vi "Main.vi"(11 "Module Admin":refnum<class "Delacor_lib_QMH_Module Admin.lvclass">) -> ()   [LabVIEW 2026, in "Replay.lvlib"]
doc: "This template is based off of the Queued Message Handler design pattern and the Queued Message Handler project template that ships with LabVIEW.\n\nThe main difference is that the queue is private to this module and communication between modules is performed via Broadcast and Request events.\n\nRequest events are wrapped in public API methods and are handled in the Event Handling Loop (EHL) of this VI. Any module can register for Broadcast events sent by this module. The EHL generates messages based on user interface actions.\n\nThe Message Handling Loop (MHL) processes messages generated by the EHL, or by other messages. The messages are string values, so new messages can be added easily to the Message Cases case structure in the MHL. Each message cluster can also provide an optional value for Message Data, which is a variant that can be converted to whatever message-specific data is required.\n_____\nBased on DQMH Dev Tools: Project Template 7.1.2.1547."
uses:
  Replay.lvlib
  <vilib>/Delacor/Delacor QMH/Libraries/Message Queue_class/Delacor_lib_QMH_Message Queue.lvclass
  Module Data--cluster.ctl
  <vilib>/Utility/miscctls.llb/LVPointTypeDef.ctl
  <vilib>/Delacor/Delacor QMH/Libraries/Message Queue_class/Delacor_lib_QMH_Enqueue Message (Single).vi
  Stop Argument--cluster.ctl
  <vilib>/Delacor/Delacor QMH/Libraries/Module Admin_class/Delacor_lib_QMH_Module Admin.lvclass
  Launcher/Launcher.lvlib
  Replay Helper Loop.ctl
  User Events Metadata.ctl
  <vilib>/Wovalab/Utilities/Helper Loop Periodic Timing/Helper Loop Periodic Timing.lvclass
panel:
  out "error out":errorcluster
  out "Status":string
  in  "Simulate MHL Error":bool
  in  "Simulate EHL Error":bool
  # "Other processes communicate with this Module via its Public API (wrappers for its Request Events).\n\nThis Module communicates with other processes via its Broadcast Events.\nAny process that wants to receive these messages can register for this module's Broadcast events."
  # "This template is for the DQMH framework. See the block diagram for more information on how to use this template."
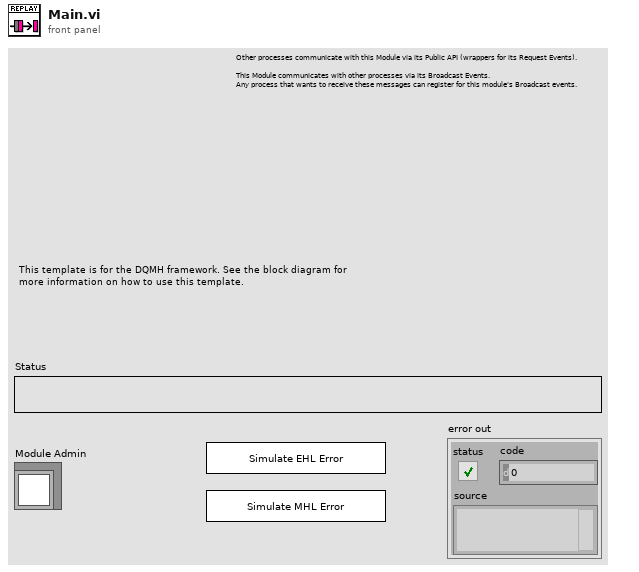
[diagram p1: front panel]
types:
  T1 = typedef "Replay.lvlib/Request Events--cluster.ctl" = cluster{"Stop Module":refnum<user-event>, "Show Panel":refnum<user-event>, "Hide Panel":refnum<user-event>, "Get Module Execution Status":refnum<user-event>, "Show Diagram":refnum<user-event>, "Set Run ID to Replay":refnum<user-event>}
  T2 = typedef "Launcher.lvlib/Broadcast Events--cluster.ctl" = cluster{"Module Did Init":refnum<user-event>, "Status Updated":refnum<user-event>, "Error Reported":refnum<user-event>, "Module Did Stop":refnum<user-event>, "Update Module Execution Status":refnum<user-event>, "Start Capture Detection Loop":refnum<user-event>, "Benchmark Started":refnum<user-event>, "Broadcast number of frames and run ID":refnum<user-event>}
  T3 = typedef "Replay.lvlib/Replay Helper Loop.ctl" = cluster{"Timeout":i32, "Run ID":string, "Replay Array Elements":string[], "User Events Metadata":T4[], "Frame Index":i32}
  T4 = typedef "User Events Metadata.ctl" = cluster{"Cursor Position X":i32, "Cursor Position Y":i32, "Left Button Click":bool, "Right Button Click":bool, "Frame Number":u32}
  T5 = typedef "Replay.lvlib/Module Data--cluster.ctl" = cluster{"Status":string}
  T6 = enum32{"invalid lock state", "Not Locked", "Locked (No Password)", "Password-protected"}
  T7 = typedef "Replay.lvlib/Stop Argument--cluster.ctl" = cluster{"Origin":string, "Exit via Stop Module Req?":bool, "Wait for Module to stop?":bool}
  T8 = typedef "LVPointTypeDef.ctl" = cluster{"Horizontal":i16, "Vertical":i16}
  T9 = enum32{"Invalid", "Standard", "Closed", "Hidden", "Minimized", "Maximized"}
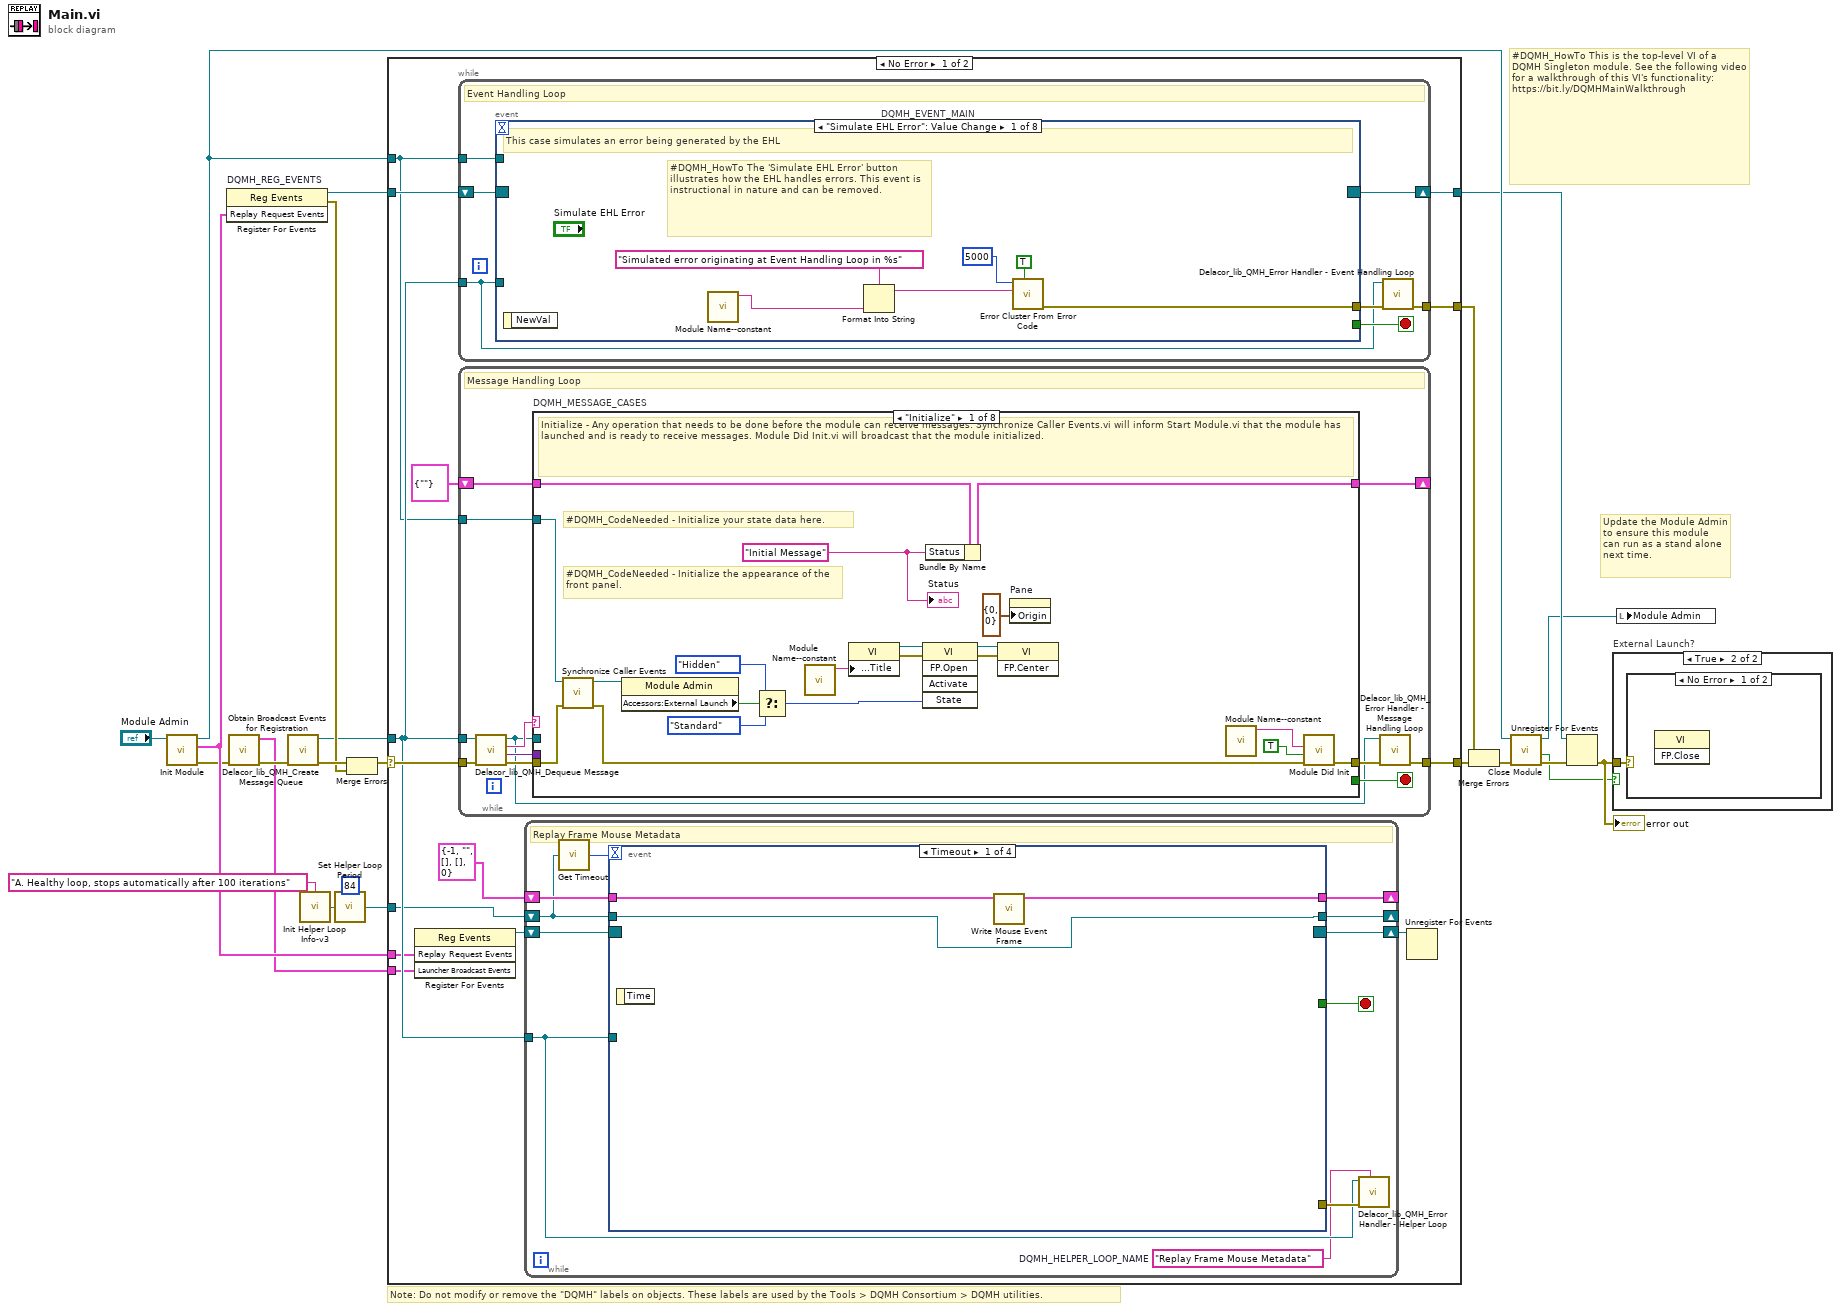
[diagram p0: block diagram]
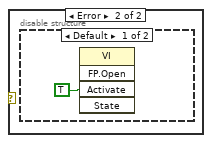
[diagram p3: hidden frame]
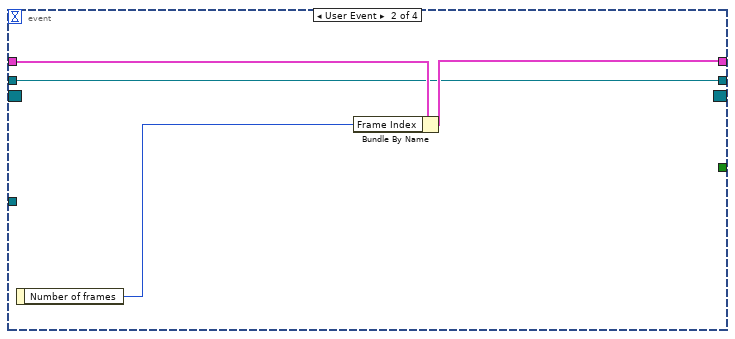
[diagram p5: hidden frame]
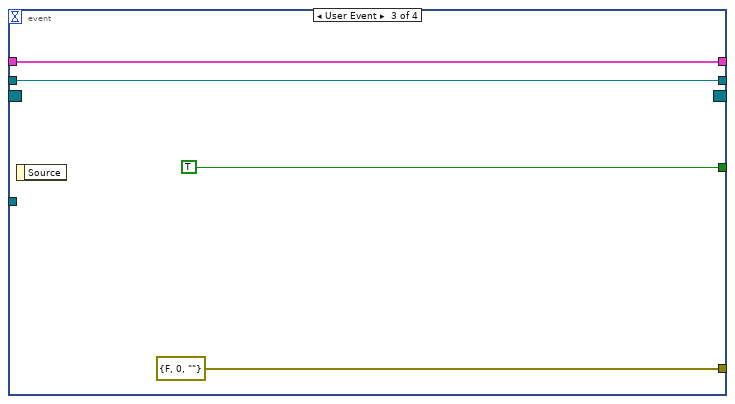
[diagram p6: hidden frame]
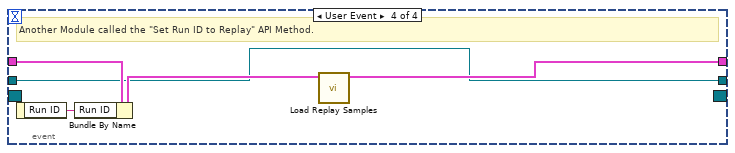
[diagram p7: hidden frame]
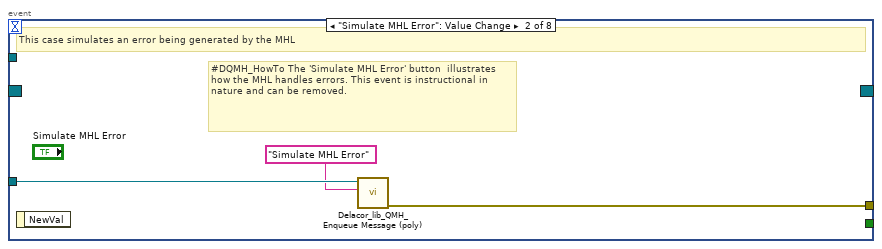
[diagram p8: hidden frame]
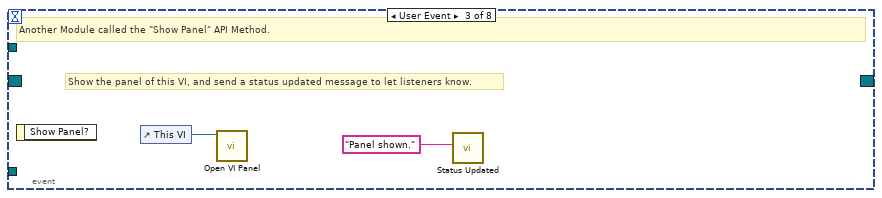
[diagram p9: hidden frame]
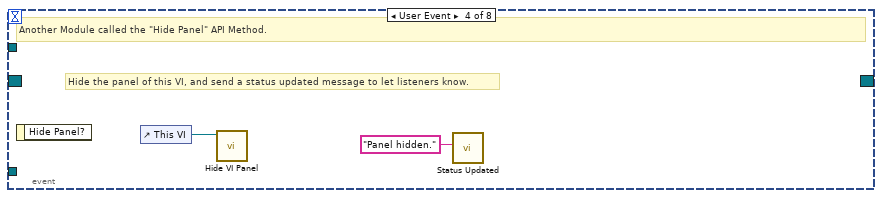
[diagram p10: hidden frame]
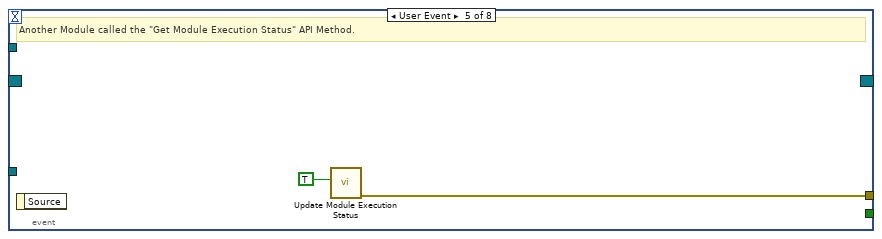
[diagram p11: hidden frame]
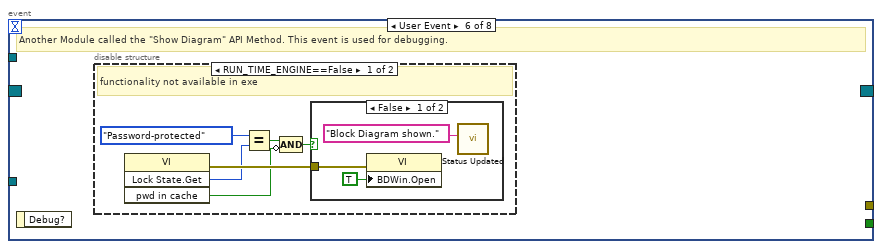
[diagram p12: hidden frame]
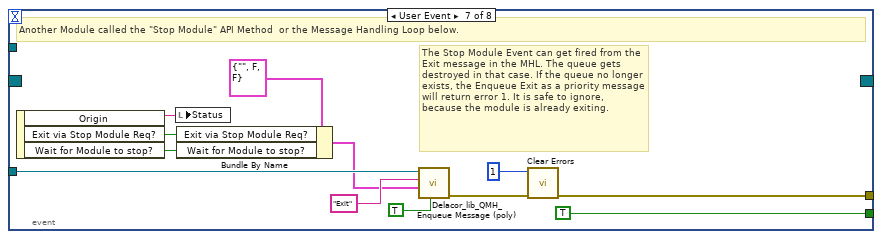
[diagram p15: hidden frame]
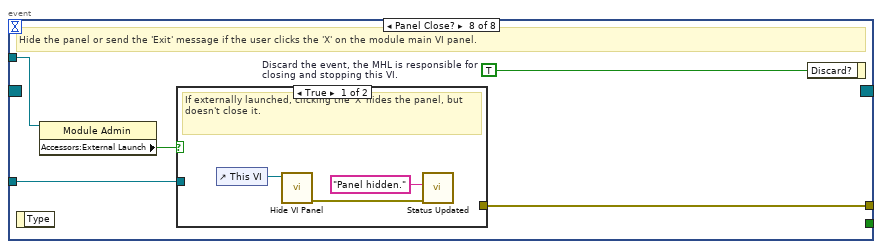
[diagram p16: hidden frame]
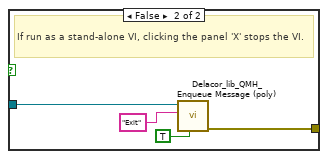
[diagram p17: hidden frame]
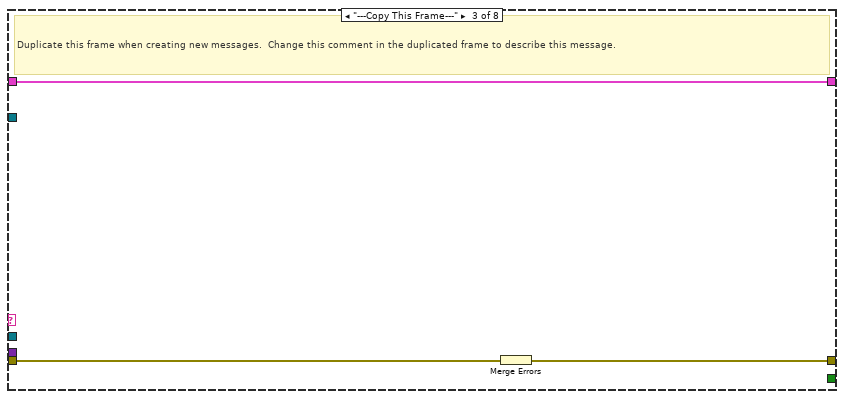
[diagram p19: hidden frame]
diagram:
  # "#DQMH_HowTo This is the top-level VI of a DQMH Singleton module. See the following video for a walkthrough of this VI's functionality: https://bit.ly/DQMHMainWalkthrough"
  # "Note: Do not modify or remove the \"DQMH\" labels on objects. These labels are used by the Tools > DQMH Consortium > DQMH utilities."
  # "Update the Module Admin to ensure this module can run as a stand alone next time."
  n1 = call "Init Module.vi"("Singleton Module Admin in"="Module Admin") -> ("error out"=w7:errorcluster, "Replay Request Events"=w8:T1, "Singleton Module Admin out"=w15:refnum<class "Delacor_lib_QMH_Module Admin.lvclass">)  [unwired: 8 in]
  n2 = register-events "DQMH_REG_EVENTS"(w8) -> (reference out=w13:refnum<event-registration>, error out=w16:errorcluster)  [unwired: 2 in]
  n3 = call "Obtain Broadcast Events for Registration.vi"("error in"=w7) -> ("error out"=w6:errorcluster, "Launcher Broadcast Events"=w5:T2)  [unwired: 8 in, 1 out]
  n4 = call <vilib>:"Delacor_lib_QMH_Create Message Queue.vi"("error in"=w6) -> ("error out"=w18:errorcluster, "Message Queue"=w12:refnum<class "Delacor_lib_QMH_Message Queue.lvclass">)  [unwired: 9 in]
  n5 = call <vilib>:"Init Helper Loop Info-v3.vi"("Loop Name (\"\": Caller VI)"="A. Healthy loop, stops automatically after 100 iterations" ("Loop Name (\"\": Caller VI)")) -> ("Helper Loop Periodic Timing"=w3:refnum<class "Helper Loop Periodic Timing.lvclass">)  [unwired: 1 in]
  n6 = call <vilib>:"Set Helper Loop Period.vi"("Period (ms)"=84, "Helper Loop Periodic Timing in"=w3) -> ("Helper Loop Periodic Timing out"=w1:refnum<class "Helper Loop Periodic Timing.lvclass">)  [unwired: 13 in]
  n7 = Merge Errors(w18, w16) -> (w17:errorcluster)
  n8 = case shown="No Error" w17 {
    selector: w17 -> [w35 w217]
    tunnel: [w37 w216] -> w23
    tunnel: [w34 w215] -> w14
    tunnel: w13 -> [w32 w215]
    tunnel: w12 -> [w31 w210]
    tunnel: [w36 _] -> w21
    tunnel: w15 -> [w30 w211]
    tunnel: w8 -> [w29 _]
    tunnel: w5 -> [w26 _]
    tunnel: w1 -> [w24 _]
    frame No Error {
      n9 = register-events ("DQMH_HELPER_REGFOREVENTS")(w29, w26) -> (reference out=w27:refnum<event-registration>)  [unwired: 2 in, 1 out]
      n10 = while {
        tunnel: w31 -> [w65]
        shift-right: [w68] -> w34
        shift-left: w32 -> [w69]
        tunnel: [w70] -> w36
        tunnel: w30 -> [w66]
        stop <- w67 stop-if-true
        # "Event Handling Loop"
        n11 = event "DQMH_EVENT_MAIN" shown="[0] \"Simulate EHL Error\": Value Change" {
          selector: w69 -> [_ _ _ _ _ _ _ _]
          dyn-events: [_ _ _ _ _ _ _ _] -> w68
          timeout: _ -> [_ _ _ _ _ _ _ _]
          tunnel: [_ _ _ _ _ _ TRUE ("Discard?") _] -> w67
          tunnel: w65 -> [_ w79 _ _ _ _ w103 w110]
          tunnel: [w77 w80 _ _ w86 _ w106 w112] -> w71
          tunnel: w66 -> [_ _ _ _ _ _ _ w109]
          event "Simulate EHL Error": Value Change {
            # "#DQMH_HowTo The 'Simulate EHL Error' button  illustrates how the EHL handles errors. This event is instructional in nature and can be removed."
            # "This case simulates an error being generated by the EHL"
            n12 = event-data() -> ()  [unwired: 1 in, 1 out]
            n13 = call "Module Name--constant.vi"() -> ("Module Name"=w74:string)  [unwired: 11 in]
            n14 = Format Into String(format string="Simulated error originating at Event Handling Loop in %s", w74) -> (resulting string=w75:string)  [unwired: 2 in, 1 out]
            n15 = call <vilib>:"Error Cluster From Error Code.vi"("show call chain? (False)"=TRUE, "error message (\"\")"=w75, "error code (0)"=5000) -> ("error out"=w77:errorcluster)  [unwired: 6 in]
          }
          event "Simulate MHL Error": Value Change {
            # "#DQMH_HowTo The 'Simulate MHL Error' button  illustrates how the MHL handles errors. This event is instructional in nature and can be removed."
            # "This case simulates an error being generated by the MHL"
            n16 = event-data() -> ()  [unwired: 1 in, 1 out]
            n17 = call-poly <vilib>:"Delacor_lib_QMH_Enqueue Message (poly).vi"("Message"="Simulate MHL Error", "Message Queue in"=w79) -> ("error out"=w80:errorcluster)  [unwired: 8 in, 1 out]
          }
          event User Event {
            # "Show the panel of this VI, and send a status updated message to let listeners know."
            # "Another Module called the \"Show Panel\" API Method."
            n18 = event-data() -> ()  [unwired: 1 in, 1 out]
            n19 = control-ref of="This VI"() -> (w82:refnum<vi>)
            n20 = call "Open VI Panel.vi"("VI"=w82) -> ()  [unwired: 10 in, 1 out]
            n21 = call "Status Updated.vi"("Status"="Panel shown." ("format string")) -> ()  [unwired: 10 in, 1 out]
          }
          event User Event {
            # "Hide the panel of this VI, and send a status updated message to let listeners know."
            # "Another Module called the \"Hide Panel\" API Method."
            n22 = event-data() -> ()  [unwired: 1 in, 1 out]
            n23 = control-ref of="This VI"() -> (w84:refnum<vi>)
            n24 = call "Hide VI Panel.vi"("VI"=w84) -> ()  [unwired: 10 in, 1 out]
            n25 = call "Status Updated.vi"("Status"="Panel hidden." ("format string")) -> ()  [unwired: 10 in, 1 out]
          }
          event User Event {
            # "Another Module called the \"Get Module Execution Status\" API Method."
            n26 = event-data() -> ()  [unwired: 1 in, 1 out]
            n27 = call "Update Module Execution Status.vi"("Running?"=TRUE) -> ("error out"=w86:errorcluster)  [unwired: 10 in]
          }
          event User Event {
            # "Another Module called the \"Show Diagram\" API Method. This event is used for debugging."
            n28 = event-data() -> ()  [unwired: 1 in, 1 out]
            n29 = disable-structure shown="RUN_TIME_ENGINE==False" {
              frame condition #0 (active) {
                # "functionality not available in exe"
                n30 = invoke on="Invoke Node" class="VI" method="Lock State.Get"() -> (error out=w92:errorcluster, "Get Lock State"=w91:T6, "pwd in cache"=w88:bool)  [unwired: 4 in, 1 out]
                n31 = Equal?(x=T6."Password-protected", y=w91) -> (x = y?=w89:bool)
                n32 = Compound Arithmetic op=AND(w89, invert w88) -> (w87:bool)
                n33 = case shown="False" w87 {
                  tunnel: w92 -> [w95 _]
                  frame False {
                    n34 = property on="Property Node" class="VI"(error in=w95, "BDWin.Open"=TRUE ("Block Diagram Window:Open")) -> ()  [unwired: 1 in, 2 out]
                    n35 = call "Status Updated.vi"("Status"="Block Diagram shown." ("format string")) -> ()  [unwired: 10 in, 1 out]
                  }
                  frame True {
                    # "Password-protected VI, and the password is not in the cache. Do not show the diagram."
                  }
                }
              }
              frame condition #1 {
              }
            }
          }
          event User Event {
            # "The Stop Module Event can get fired from the Exit message in the MHL. The queue gets destroyed in that case. If the queue no longer exists, the Enqueue Exit as a priority message will return error 1. It is safe to ignore, because the module is already exiting."
            # "Another Module called the \"Stop Module\" API Method  or the Message Handling Loop below."
            n36 = event-data() -> ("Origin"=w102:string, "Exit via Stop Module Req?"=w98:bool, "Wait for Module to stop?"=w97:bool)  [unwired: 1 in]
            n37 = local write "Status"(w102) -> ()
            n38 = Bundle By Name(cluster=T7 {"Origin"="", "Exit via Stop Module Req?"=FALSE, "Wait for Module to stop?"=FALSE} ("Stop Argument"), "Exit via Stop Module Req?"=w98, "Wait for Module to stop?"=w97) -> (w96:T7)
            n39 = call-poly <vilib>:"Delacor_lib_QMH_Enqueue Message (poly).vi"("Priority Message? (F)"=TRUE, "Message Data"=w96, "Message"="Exit", "Message Queue in"=w103) -> ("error out"=w107:errorcluster)  [unwired: 6 in, 1 out]
            n40 = call <vilib>:"Clear Errors.vi"("error in (no error)"=w107, "specific error code to clear (0: all)"=1) -> ("error out"=w106:errorcluster)  [unwired: 4 in, 1 out]
          }
          event Panel Close? {
            w111 = TRUE  # Discard the event, the MHL is responsible for closing and stopping this VI.
            # "Hide the panel or send the 'Exit' message if the user clicks the 'X' on the module main VI panel."
            n41 = event-data() -> ()  [unwired: 1 in, 1 out]
            n42 = property on="Property Node" class="Module Admin"(reference=w109) -> ("Accessors:External Launch"=w108:bool)  [unwired: 1 in, 2 out]
            n43 = case shown="True" w108 {
              tunnel: w110 -> [_ w118]
              tunnel: [_ w119] -> w112
              frame True {
                # "If externally launched, clicking the 'X' hides the panel, but doesn't close it."
                n44 = control-ref of="This VI"() -> (w115:refnum<vi>)
                n45 = call "Hide VI Panel.vi"("VI"=w115) -> ("error out"=w113:errorcluster)  [unwired: 10 in]
                n46 = call "Status Updated.vi"("error in"=w113, "Status"="Panel hidden." ("format string")) -> ()  [unwired: 9 in, 1 out]
              }
              frame False {
                # "If run as a stand-alone VI, clicking the panel 'X' stops the VI."
                n47 = call-poly <vilib>:"Delacor_lib_QMH_Enqueue Message (poly).vi"("Priority Message? (F)"=TRUE, "Message"="Exit", "Message Queue in"=w118) -> ("error out"=w119:errorcluster)  [unwired: 7 in, 1 out]
              }
            }
            n48 = event-data ("Event Filter Node")("Discard?"=w111) -> ()  [unwired: 1 in, 1 out]
          }
        }
        n49 = call-dynamic "Delacor_lib_QMH_Error Handler - Event Handling Loop.vi"("error in"=w71, "Message Queue in"=w65) -> ("dup error in"=w70:errorcluster)  [unwired: 8 in, 1 out]
      }
      n50 = while {
        tunnel: w31 -> [w120]
        shift-right: [w128] -> _
        shift-left: T5 {"Status"=""} ("Data Cluster") -> [w129]
        tunnel: w35 -> [w131]
        tunnel: [w123] -> w37
        tunnel: w30 -> [w124]
        stop <- w127 stop-if-true
        # "Message Handling Loop"
        n51 = call-dynamic "Delacor_lib_QMH_Dequeue Message.vi"("error in"=w131, "Message Queue in"=w120) -> ("error out"=w130:errorcluster, "Message Data"=w125:variant, "Message"=w126:string, "Message Queue out"=w121:refnum<class "Delacor_lib_QMH_Message Queue.lvclass">)  [unwired: 6 in]
        n52 = case "DQMH_MESSAGE_CASES" shown="\"Initialize\"" w126 {
          selector: w126 -> [_ _ _ _ _ _ _ w205]
          tunnel: w121 -> [_ _ _ _ _ w171 w193 _]
          tunnel: w130 -> [w149 w153 w156 w158 w167 w178 w199 w208]
          tunnel: [w147 w153 w155 w158 w166 w174 w194 w209] -> w122
          tunnel: w129 -> [w138 w152 w154 w157 w164 w173 w192 w206]
          tunnel: [w137 w152 w154 w157 w164 w173 w192 w206] -> w128
          tunnel: [_ _ _ _ _ _ w191 _] -> w127
          tunnel: w125 -> [_ _ _ _ _ w172 w190 _]
          tunnel: w124 -> [w139 _ _ _ _ w170 w185 _]
          frame "Initialize" {
            w133 = "Initial Message" ("Initial Message")
            # "#DQMH_CodeNeeded - Initialize the appearance of the front panel."
            # "#DQMH_CodeNeeded - Initialize your state data here."
            # "Initialize - Any operation that needs to be done before the module can receive messages. Synchronize Caller Events.vi will inform Start Module.vi that the module has launched and is ready to receive messages. Module Did Init.vi will broadcast that the module initialized."
            n53 = call "Synchronize Caller Events.vi"("error in"=w149, "Singleton Module Admin in"=w139) -> ("error out"=w148:errorcluster, "Singleton Module Admin out"=w134:refnum<class "Delacor_lib_QMH_Module Admin.lvclass">)  [unwired: 8 in]
            n54 = property on="Property Node" class="Module Admin"(reference=w134) -> ("Accessors:External Launch"=w143:bool)  [unwired: 1 in, 2 out]
            n55 = Select(t=T9."Hidden" ("State"), s=w143, f=T9."Standard" ("State")) -> (s? t:f=w140:T9)
            n56 = call "Module Name--constant.vi"() -> ("Module Name"=w146:string)  [unwired: 11 in]
            n57 = property on="Property Node" class="VI"("Front Panel.Title"=w146) -> (reference out=w145:refnum<vi>, error out=w151:errorcluster)  [unwired: 2 in]
            n58 = invoke on="Invoke Node" class="VI" method="FP.Open"(reference=w145, error in=w151, "State"=w140) -> (reference out=w144:refnum<vi>, error out=w150:errorcluster)  [unwired: 2 in, 3 out]
            n59 = Bundle By Name(cluster=w138, "Status"=w133) -> (w137:T5)
            n60 = invoke on="Invoke Node" class="VI" method="FP.Center"(reference=w144, error in=w150) -> ()  [unwired: 1 in, 3 out]
            n61 = property on="Pane" class="Pane"("Origin"=T8 {"Horizontal"=0, "Vertical"=0}) -> ()  [unwired: 2 in, 2 out]
            n62 = call "Module Name--constant.vi"() -> ("Module Name"=w135:string)  [unwired: 11 in]
            n63 = call "Module Did Init.vi"("error in"=w148, "Initialized?"=TRUE, "Origin"=w135) -> ("error out"=w147:errorcluster)  [unwired: 8 in]
            "Status" <- w133
          }
          frame "---Module Specific---" {
            # "Separator -- The following cases handle messages specific to this Module."
          }
          frame "---Copy This Frame---" {
            # "Duplicate this frame when creating new messages.  Change this comment in the duplicated frame to describe this message."
            n64 = Merge Errors(w156) -> (w155:errorcluster)
          }
          frame "---Exit and Error Handling---" {
            # "Separator - The following cases handle errors and exit messages."
          }
          frame "Simulate MHL Error" {
            # "#DQMH_HowTo The 'Simulate MHL Error' button  illustrates how the MHL handles errors. This event is instructional in nature and can be removed."
            # "Simulate an error occurring at the MHL"
            n65 = call "Module Name--constant.vi"() -> ("Module Name"=w160:string)  [unwired: 11 in]
            n66 = Format Into String(format string="Simulated error originating at Message Handling Loop in %s", w160) -> (resulting string=w161:string)  [unwired: 2 in, 1 out]
            n67 = call <vilib>:"Error Cluster From Error Code.vi"("show call chain? (False)"=TRUE, "error message (\"\")"=w161, "error code (0)"=5001) -> ("error out"=w165:errorcluster)  [unwired: 6 in]
            n68 = Merge Errors(w167, w165) -> (w166:errorcluster)
          }
          frame "Error" {
            # "#DQMH_CodeRecommended - If the module is running in standalone mode (External Launch = FALSE), this code will pop up an error dialog and call the 'Exit' message if an error occurs. Add more fine-grained error management here."
            # "Error - Check the error message data and respond accordingly. This message is sent by the \"Error Handler\" VIs at the end of each loop in this application."
            n69 = property on="Property Node" class="Module Admin"(reference=w170) -> ("Accessors:External Launch"=w169:bool)  [unwired: 1 in, 2 out]
            n70 = Variant To Data(error in=w178, type=errorcluster {"status"=FALSE, "code"=0, "source"=""} ("error constant"), Variant=w172) -> (data=w168:errorcluster, error out=w176:errorcluster)
            n71 = local write "error out"(w168) -> ()
            n72 = call "Error Reported.vi"("Error"=w168) -> ()  [unwired: 10 in, 1 out]
            n73 = case shown="False" w169 {
              tunnel: [w183 _] -> w175
              tunnel: w171 -> [w181 _]
              tunnel: w168 -> [w182 _]
              frame False {
                n74 = disable-structure shown="Default" {
                  disable-tunnel: w182 -> [w184 _]
                  frame condition #0 (active) {
                    # "If the module is running standalone, then pop up an error dialog and call the \"Exit\" message."
                    n75 = call <vilib>:"Simple Error Handler.vi"("error in (no error)"=w184) -> ()  [unwired: 4 in, 5 out]
                  }
                  frame condition #1 {
                    # "To prevent the Simple Error Handler VI from being loaded (e.g. when deploying to a Real-Time target), add the Conditional Disable Symbol \"DQMH_Disable_SEH\" to your project and set it to TRUE."
                  }
                }
                n76 = call-poly <vilib>:"Delacor_lib_QMH_Enqueue Message (poly).vi"("Priority Message? (F)"=TRUE, "Message"="Exit", "Message Queue in"=w181) -> ("error out"=w183:errorcluster)  [unwired: 7 in, 1 out]
              }
              frame True {
                # "If the module was launched externally, calling the Error Reported broadcast VI is the only action performed by the \"Error\" message. The module's caller can then process the error appropriately."
              }
            }
            n77 = Merge Errors(w176, w175) -> (w174:errorcluster)
          }
          frame "Exit" {
            w189 = 91  # 91: not all Exit messages will have an argument
            w191 = TRUE  # Stop the VI
            # "Release the message queue reference"
            # "#DQMH_CodeNeeded - Add any required cleanup code here."
            # "Exit - Exit the application."
            n78 = Variant To Data(error in=w199, type=T7 {"Origin"="", "Exit via Stop Module Req?"=FALSE, "Wait for Module to stop?"=FALSE} ("Stop Argument"), Variant=w190) -> (data=w187:T7, error out=w196:errorcluster)
            n79 = call <vilib>:"Clear Errors.vi"("error in (no error)"=w196, "specific error code to clear (0: all)"=w189) -> ("error out"=w198:errorcluster)  [unwired: 4 in, 1 out]
            n80 = control-ref of="This VI"() -> (w186:refnum<vi>)
            n81 = call-dynamic "Delacor_lib_QMH_Release Message Queue.vi"("error in"=w198, "Message Queue"=w193) -> ("error out"=w197:errorcluster)  [unwired: 9 in]
            n82 = call "Handle Exit.vi"("Stop Argument"=w187, "Admin in"=w185, "VI reference"=w186) -> ("error out"=w195:errorcluster)  [unwired: 7 in, 1 out]
            n83 = Merge Errors(w197, w195) -> (w194:errorcluster)
            n84 = call "Error Reported.vi"("Error"=w194) -> ()  [unwired: 10 in, 1 out]
          }
          frame Default {
            # "'Default' case only runs if there is a message that isn't defined in any of the other cases.  Output a programming error."
            n85 = call "Module Name--constant.vi"() -> ("Module Name"=w204:string)  [unwired: 11 in]
            n86 = Format Into String(format string="The invalid message string \"%s\" was received in the Message Handling Loop for module \"%s\".", w205, w204) -> (resulting string=w200:string)  [unwired: 2 in, 1 out]
            n87 = call <vilib>:"Error Cluster From Error Code.vi"("show call chain? (False)"=TRUE, "error message (\"\")"=w200, "error code (0)"=1) -> ("error out"=w207:errorcluster)  [unwired: 6 in]
            n88 = Merge Errors(w208, w207) -> (w209:errorcluster)
          }
        }
        n89 = call-dynamic "Delacor_lib_QMH_Error Handler - Message Handling Loop.vi"("error in"=w122, "Message Queue in"=w121) -> ("dup error in"=w123:errorcluster)  [unwired: 8 in, 1 out]
      }
      n90 = while "DQMH_HELPER_LOOP" {
        shift-right: [w48] -> _
        shift-left: T3 {"Timeout"=-1, "Run ID"="", "Replay Array Elements"=[], "User Events Metadata"=[], "Frame Index"=0} ("Replay Helper Loop") -> [w41]
        shift-right: [w46] -> w28
        shift-left: w27 -> [w47]
        tunnel: w31 -> [w43]
        shift-right: [w38] -> _
        shift-left: w24 -> [w39]
        stop <- w45 stop-if-true
        w42 = "Replay Frame Mouse Metadata"  # DQMH_HELPER_LOOP_NAME
        # "Replay Frame Mouse Metadata"
        n91 = call <vilib>:"Get Timeout.vi"("Helper Loop Periodic Timing"=w39) -> ("Timeout (ms)"=w40:i32)  [unwired: 12 in, 2 out]
        n92 = event "DQMH_HELPER_EVENT_STRUCTURE" shown="[0] Timeout" {
          selector: w47 -> [_ _ _ _]
          dyn-events: [_ _ _ _] -> w46
          timeout: w40 -> [_ _ _ _]
          tunnel: w41 -> [w51 w55 w59 w64]
          tunnel: [w50 w54 w59 w61] -> w48
          tunnel: [_ _ TRUE _] -> w45
          tunnel: [_ _ errorcluster {"status"=FALSE, "code"=0, "source"=""} ("error constant") _] -> w44
          tunnel: w43 -> [_ _ _ _]
          tunnel: w39 -> [w49 w53 w56 w60]
          tunnel: [w49 w53 w56 w60] -> w38
          event Timeout {
            n93 = event-data() -> ()  [unwired: 1 in, 1 out]
            n94 = call "Write Mouse Event Frame.vi"("Replay Helper Loop In"=w51) -> ("Replay Helper Loop Out"=w50:T3)  [unwired: 10 in]
          }
          event User Event {
            n95 = event-data() -> ("Number of frames"=w52:u32)  [unwired: 1 in]
            n96 = Bundle By Name(cluster=w55, "Frame Index"=w52) -> (w54:T3)
          }
          event User Event {
            n97 = event-data() -> ()  [unwired: 1 in, 1 out]
          }
          event User Event {
            # "Another Module called the \"Set Run ID to Replay\" API Method."
            n98 = event-data() -> ("Run ID"=w63:string)  [unwired: 1 in]
            n99 = Bundle By Name(cluster=w64, "Run ID"=w63) -> (w62:T3)
            n100 = call "Load Replay Samples.vi"("Replay Helper Loop In"=w62) -> ("Replay Helper Loop Out"=w61:T3)  [unwired: 10 in]
          }
        }
        n101 = call-dynamic "Delacor_lib_QMH_Error Handler - Helper Loop.vi"("Error Debug"=w42, "error in"=w44, "Message Queue in"=w43) -> ()  [unwired: 7 in, 2 out]
      }
      n102 = Unregister For Events(event registration refnum=w28) -> ()  [unwired: 1 in, 1 out]
    }
    frame Error {
      # "Synchronize Caller Events.vi will inform Start Module.vi that the module has launched and will let the code calling Start Module.vi register for broadcasts and would permit the caller receive the broadcast that an error occurred at launch time."
      n103 = call-dynamic "Delacor_lib_QMH_Release Message Queue.vi"("error in"=w217, "Message Queue"=w210) -> ("error out"=w216:errorcluster)  [unwired: 9 in]
      n104 = call "Synchronize Caller Events.vi"("Singleton Module Admin in"=w211) -> ("error out"=w218:errorcluster)  [unwired: 9 in, 1 out]
      n105 = call "Module Name--constant.vi"() -> ("Module Name"=w214:string)  [unwired: 11 in]
      n106 = Format Into String(format string="An error occurred during initialization. %s is no longer running.", w214) -> (resulting string=w212:string)  [unwired: 2 in, 1 out]
      n107 = Merge Errors(w216, w218) -> (w219:errorcluster)
      n108 = call "Error Reported.vi"("Additional Information"=w212, "Error"=w219) -> ()  [unwired: 9 in, 1 out]
    }
  }
  n109 = Merge Errors(w21, w23) -> (w20:errorcluster)
  n110 = call "Close Module.vi"("error in"=w20, "Module Admin in"=w15) -> ("error out"=w22:errorcluster, "External Launch"=w9:bool, "Module Admin out"=w10:refnum<class "Delacor_lib_QMH_Module Admin.lvclass">)  [unwired: 7 in]
  n111 = Unregister For Events(event registration refnum=w14, error in=w22) -> (error out=w19:errorcluster)
  "error out" <- w19
  n112 = case "External Launch?" shown="True" w9 {
    tunnel: w19 -> [_ w220]
    frame False {
    }
    frame True {
      n113 = case shown="No Error" w220 {
        frame No Error {
          n114 = invoke on="Invoke Node" class="VI" method="FP.Close"() -> ()  [unwired: 3 in, 3 out]
        }
        frame Error {
          n115 = disable-structure shown="Default" {
            frame condition #0 (active) {
              n116 = invoke class="VI" method="FP.Open"("Activate"=TRUE ("Activate?")) -> ()  [unwired: 4 in, 5 out]
            }
            frame condition #1 {
              # "Don't show panel on error if running inside a built EXE."
            }
          }
        }
      }
    }
  }
  n117 = local write "Module Admin"(w10) -> ()
